vi "practice06_led_control.vi"() -> ()   [LabVIEW 2025]
uses:
  <vilib>/Instr/_visa.llb/VISA Configure Serial Port (Instr).vi
panel:
  out "Digitos binarios":string
  out "Numero":u32
  in  "Dig 9":bool
  in  "Pin 2":bool
  in  "Pin 3":bool
  in  "Pin 4":bool
  in  "Pin 5":bool
  in  "Pin 6":bool
  in  "Pin 7":bool
  in  "Dig 8":bool
  in  "stop":bool
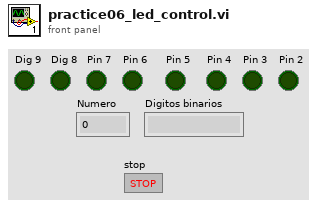
[diagram p1: front panel]
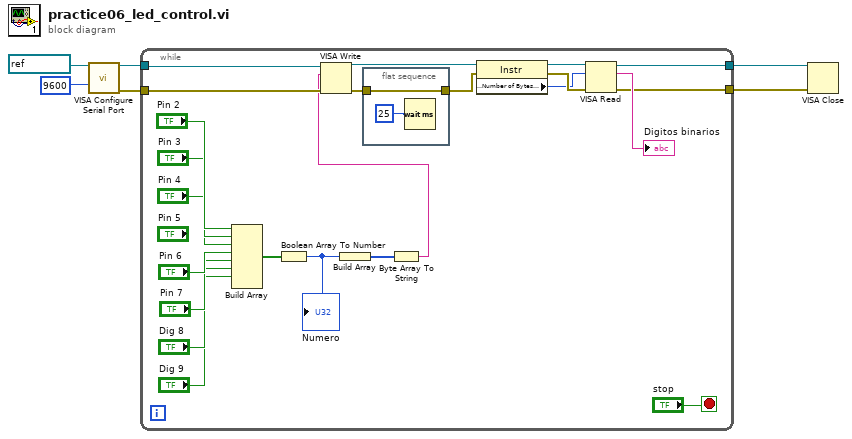
[diagram p0: block diagram]
diagram:
  n1 = call-poly "VISA Configure Serial Port"("VISA resource name"=refnum<visa-resource-name> "COM3", "parity (0:none)"=9600) -> ("VISA resource name out"=w4:refnum<visa-resource-name>, "error out"=w3:errorcluster)  [unwired: 12 in]
  n2 = while {
    tunnel: w4 -> [w26]
    tunnel: w3 -> [w25]
    tunnel: [w8] -> w2
    tunnel: [w7] -> w1
    stop <- "stop" stop-if-true
    n3 = Build Array("Pin 2", "Pin 3", "Pin 4", "Pin 6", "Pin 7", "Dig 8", "Dig 9") -> (w12:bool[])  [unwired: 1 in]
    n4 = Boolean Array To Number(Boolean array=w12) -> (number=w10:u32)
    "Numero" <- w10
    n5 = Build Array(w10) -> (w11:u32[])
    n6 = flat-sequence {
      tunnel: w23 -> [w31]
      tunnel: [w31] -> w22
      frame #0 {
        n7 = Wait (ms)(milliseconds to wait=u32 25) -> ()  [unwired: 1 out]
      }
    }
    n8 = Byte Array To String(unsigned byte array=w11) -> (string=w20:string)
    n9 = VISA Write(VISA resource name=w26, write buffer=w20, error in (no error)=w25) -> (VISA resource name out=w24:refnum<visa-resource-name>, error out=w23:errorcluster)  [unwired: 1 out]
    n10 = property class="Instr"(reference=w24, error in=w22) -> (reference out=w28:refnum<visa-resource-name>, error out=w27:errorcluster, "Serial Settings:Number of Bytes at Serial Port"=w21:u32)
    n11 = VISA Read(VISA resource name=w28, byte count=w21, error in (no error)=w27) -> (VISA resource name out=w8:refnum<visa-resource-name>, read buffer=→"Digitos binarios":string, error out=w7:errorcluster)  [unwired: 1 out]
  }
  n12 = VISA Close(VISA resource name=w2, error in (no error)=w1) -> ()  [unwired: 1 out]
